vi "Measurement Logic.vi"() -> ()   [LabVIEW 2024, in "Frequency Response (Discrete Sweep).lvlib"]
uses:
  Frequency Response (Discrete Sweep).lvlib
  <vilib>/Plug-In SDKs/Measurements/Measure Call Context/Measure Call Context.lvclass
  Measurement Configuration.ctl
  Measurement Results.ctl
  <vilib>/gRPC/Generated APIs/ni/protobuf/types/RPC Messages/ni_protobuf_types_DoubleXYData.ctl
  C:/Program Files/NI/LVAddons/nisvt/1/examples/Sound and Vibration/Audio Measurements/subVIs/sv_AO Channel Configuration.ctl
  C:/Program Files/NI/LVAddons/nisvt/1/examples/Sound and Vibration/Audio Measurements/subVIs/sv_AI Channel Configuration.ctl
  <vilib>/addons/_NISVFA/_Shared subVIs/Controls/svc_Window.ctl
  <vilib>/addons/_NISVFA/_Generation/Signal Generation/SV Signal/SV Signal.lvclass/SV Signal.ctl
  <vilib>/addons/Sound and Vibration/svt_Level/SVL AC & DC Level (Time) (1 Ch).vi
  <vilib>/addons/_NISVFA/_Shared subVIs/Common/SV Append Data (1 Ch) (DBL).vi
  <vilib>/addons/_NISVFA/_Shared subVIs/Common/SV Append Data (N Ch) (DBL).vi
  <extravilib>/ChannelInstances/High Speed Stream-a[.](wfm(dbl))/_Read For Replicate.vi
  <vilib>/addons/_NISVFA/_Shared subVIs/Common/svc_Get SV Channel Info.vi
  <vilib>/Analysis/baseanly.llb/Mean.vi
  <vilib>/Analysis/baseanly.llb/Mean (DBL).vi
  <vilib>/addons/_NISVFA/_Shared subVIs/Windowing/svfa_Scaled Time Domain Window (Array).vi
  <extravilib>/ChannelInstances/Tag-bool/Write.vi
  <vilib>/DAQmx/read.llb/DAQmx Read.vi
  <vilib>/DAQmx/read.llb/DAQmx Read (Analog 1D Wfm NChan NSamp Duration).vi
  <extravilib>/ChannelInstances/High Speed Stream-a[.](wfm(dbl))/Write.vi
  <vilib>/DAQmx/write.llb/DAQmx Write.vi
  <vilib>/DAQmx/write.llb/DAQmx Write (Analog Wfm 1Chan NSamp).vi
  C:/Program Files/NI/LVAddons/nisvt/1/examples/Sound and Vibration/Audio Measurements/subVIs/sv_Synchronization Gatekeeper.vi
  <vilib>/Utility/error.llb/Clear Errors.vi
  C:/Program Files/NI/LVAddons/nisvt/1/examples/Sound and Vibration/Audio Measurements/subVIs/sv_Align and Parse for Stimulus Response.vi
  C:/Program Files/NI/LVAddons/nisvt/1/examples/Sound and Vibration/Audio Measurements/subVIs/sv_Synchronize Acquisition and Generation.vi
  C:/Program Files/NI/LVAddons/nisvt/1/examples/Sound and Vibration/Audio Measurements/subVIs/sv_Synchronize DSA AI and AO Tasks.vi
  <vilib>/addons/_NISVFA/_Shared subVIs/Common/svc_Unit Label to Engineering Units.vi
  <vilib>/addons/_NISVFA/_Shared subVIs/Common/svc_Engineering Units to Unit Label.vi
  <vilib>/addons/_NISVFA/_Spectrum Processing/subVIs/svfa_Spectrum Info Window to windowTd Type Def.vi
  <vilib>/Analysis/4window.llb/Force Window.vi
  <vilib>/Analysis/4window.llb/Force Window (DBL).vi
  <vilib>/Analysis/4window.llb/Exponential Window.vi
  <vilib>/Analysis/4window.llb/Exponential Window (DBL).vi
  <extravilib>/ChannelInstances/Tag-bool/Read With Abort.vi
  <extravilib>/ChannelInstances/Tag-bool/Write With Abort.vi
  C:/Program Files/NI/LVAddons/nisvt/1/examples/Sound and Vibration/Audio Measurements/subVIs/sv_Prepare Acquired Waveforms for Parsing.vi
  C:/Program Files/NI/LVAddons/nisvt/1/examples/Sound and Vibration/Audio Measurements/subVIs/sv_Timing for Stimulus Response Tasks.vi
  <vilib>/addons/_NISVFA/_Generation/Signal Generation/SV Signal/Read Total Samples.vi
  <vilib>/addons/_NISVFA/_Generation/Signal Generation/SV Signal/Write Leading Synchronization Pulse Enable.vi
  C:/Program Files/NI/LVAddons/nisvt/1/examples/Sound and Vibration/Audio Measurements/subVIs/sv_Synchronization Keymaster.vi
  C:/Program Files/NI/LVAddons/nisvt/1/examples/Sound and Vibration/Audio Measurements/subVIs/sv_Get Reference Clock.vi
  C:/Program Files/NI/LVAddons/nisvt/1/examples/Sound and Vibration/Audio Measurements/subVIs/sv_Synchronization Keymaster_GO.vi
  <extravilib>/ChannelInstances/Tag-c(ref(UserDefinedRefnumTag),t'Rendezvous RefNum')/Read With Abort.vi
  C:/Program Files/NI/LVAddons/nisvt/1/examples/Sound and Vibration/Audio Measurements/subVIs/sv_Align Waveforms by Leading Sync Pulse.vi
  <vilib>/addons/_NISVFA/_Generation/Signal Generation/SV Signal/Read Synchronization Pulse Waveform.vi
  <vilib>/addons/_NISVFA/_Shared subVIs/Common/svc_Check for Waveform Parameter Continuity (N Ch).vi
  C:/Program Files/NI/LVAddons/nisvt/1/examples/Sound and Vibration/Audio Measurements/subVIs/sv_Append Virtual Reference.vi
  <vilib>/addons/_NISVFA/_Generation/Signal Generation/SV Signal/Calculate Number of Remaining Samples.vi
  <extravilib>/ChannelInstances/Tag-c(ref(UserDefinedRefnumTag),t'Rendezvous RefNum')/Write.vi
  C:/Program Files/NI/LVAddons/nisvt/1/examples/Sound and Vibration/Audio Measurements/subVIs/sv_Measure Delay for Active and Idle Channels.vi
  <vilib>/addons/_NISVFA/_Generation/Signal Generation/SV Signal/Read Leading Synchronization Pulse Enable.vi
  <vilib>/addons/_NISVFA/_Generation/Signal Generation/SV Signal/Read Trailing Synchronization Pulse Enable.vi
  <vilib>/addons/_NISVFA/_Shared subVIs/Common/svc_Check for Waveform Parameter Continuity (no state).vi
  <vilib>/addons/_NISVFA/_Shared subVIs/Common/sv_Get NI Property Name String.vi
  <extravilib>/ChannelInstances/Tag-c(ref(UserDefinedRefnumTag),t'Rendezvous RefNum')/Write With Abort.vi
  <vilib>/addons/Sound and Vibration/svt_Calibration/SV Measure Delay and Polarity and Coherence (Nx1).vi
  C:/Program Files/NI/LVAddons/nisvt/1/examples/Sound and Vibration/Audio Measurements/subVIs/sv_Assign Delay to Idle Channels.vi
  <vilib>/addons/Sound and Vibration/svt_Calibration/SV Measure Delay and Polarity and Coherence.vi
  <vilib>/Analysis/_algsub.llb/Vector Norm.vi
  <vilib>/Analysis/_algsub.llb/Real Vector Norm.vi
  <vilib>/addons/_NISVFA/_Shared subVIs/Common/SV Get Data Subset.vi
  <vilib>/addons/_NISVFA/_Shared subVIs/Common/svc_Get Array Subset (Index).vi
  <vilib>/addons/_NISVFA/_Shared subVIs/Common/svc_Coerce Index and Length.vi
  <vilib>/addons/_NISVFA/_Shared subVIs/Common/svc_Conditional Merge Error.vi
  <vilib>/addons/_NISVFA/_Generation/Signal Generation/SV Discrete Sweep/SV Discrete Sweep.lvclass
  <extravilib>/ChannelInstances/Tag-bool/Instantiate.vi
  <extravilib>/ChannelInstances/High Speed Stream-a[.](wfm(dbl))/Instantiate.vi
  <vilib>/addons/_NISVFA/_Generation/Signal Generation/SV Discrete Sweep/Configure Frequency Sweep at Constant Amplitude.vi
  <vilib>/addons/_NISVFA/_Generation/Signal Generation/SV Signal/Write Ramp Parameters.vi
  <vilib>/addons/_NISVFA/_Generation/Signal Generation/SV Function/Write Pre-Measurement Settling Cycles.vi
  <vilib>/addons/_NISVFA/_Generation/Signal Generation/SV Function/Write Measurement Cycles.vi
  <vilib>/addons/_NISVFA/_Generation/Signal Generation/SV Signal/Write Measurement Duration.vi
  <extravilib>/ChannelInstances/High Speed Stream-a[.](wfm(dbl))/)Channel.vi
  <extravilib>/ChannelInstances/High Speed Stream-a[.](wfm(dbl))/Abort Signal/Init Signal.vi
  <vilib>/addons/_NISVFA/_Shared subVIs/Common/svc_Get Window Info.vi
  <vilib>/Analysis/0measdsp.llb/Scaled Time Domain Window.vi
  <vilib>/Analysis/0measdsp.llb/Scaled Time Domain Window (DBL).vi
  <vilib>/Utility/error.llb/Error Cluster From Error Code.vi
  <vilib>/Analysis/baseanly.llb/Std Deviation and Variance.vi
  <vilib>/addons/_NISVFA/_Shared subVIs/Common/svc_Caller VI Returned in Error Source.vi
  <vilib>/addons/Sound and Vibration/svt_Single Tone Measurements/SVT Gain and Phase (Time).vi
  <vilib>/addons/Sound and Vibration/svt_Distortion/SVT THD+N (Frequency) (1 Ch).vi
  <vilib>/addons/Sound and Vibration/svt_Distortion/SVT THD and Harmonic Components (Frequency) (1 Ch).vi
  <vilib>/addons/_NIFileIO/SV TDMS Write Waveform (N Ch).vi
  <extravilib>/ChannelInstances/Tag-bool/EndpointRead.vi
  <extravilib>/ChannelInstances/Tag-bool/Endpoint.vi
  <extravilib>/ChannelInstances/Tag-c(ref(UserDefinedRefnumTag),t'Rendezvous RefNum')/Instantiate.vi
  C:/Program Files/NI/LVAddons/nisvt/1/examples/Sound and Vibration/Audio Measurements/subVIs/sv_Configure AI Task.vi
  C:/Program Files/NI/LVAddons/nisvt/1/examples/Sound and Vibration/Audio Measurements/subVIs/sv_Configure AO Task.vi
  <vilib>/addons/_NISVFA/_Generation/Signal Generation/SV Signal/Read Sample Rate.vi
  <vilib>/addons/_NISVFA/_Generation/Signal Generation/SV Signal/Read Generation State.vi
  <vilib>/addons/_NISVFA/_Generation/Signal Generation/SV Signal/Read System Timing Model.vi
  <vilib>/DAQmx/configure/timing.llb/DAQmx Timing.vi
  <vilib>/DAQmx/configure/timing.llb/DAQmx Timing (Sample Clock).vi
  <vilib>/addons/_NISVFA/_Generation/Signal Generation/SV Signal/Write Sample Rate.vi
  <vilib>/DAQmx/configure/task.llb/DAQmx Stop Task.vi
  C:/Program Files/NI/LVAddons/nisvt/1/examples/Sound and Vibration/Audio Measurements/subVIs/sv_Get Bus Type and Product Type.vi
  <vilib>/DAQmx/configure/task.llb/DAQmx Control Task.vi
  <vilib>/Utility/rendezvs.llb/Create Rendezvous.vi
  <vilib>/Utility/rendezvs.llb/Wait at Rendezvous.vi
  <extravilib>/ChannelInstances/Tag-c(ref(UserDefinedRefnumTag),t'Rendezvous RefNum')/Endpoint.vi
  <vilib>/addons/Sound and Vibration/svt_DAQmx/subVIs/svl_Get Terminal Name with Device Prefix.vi
  <vilib>/DAQmx/configure/trigger.llb/DAQmx Trigger.vi
  <vilib>/DAQmx/configure/trigger.llb/DAQmx Start Trigger (Digital Edge).vi
  <vilib>/DAQmx/configure/task.llb/DAQmx Start Task.vi
  <extravilib>/ChannelInstances/Tag-c(ref(UserDefinedRefnumTag),t'Rendezvous RefNum')/EndpointRead.vi
  <vilib>/Utility/rendezvs.llb/Destroy Rendezvous.vi
  <vilib>/DAQmx/miscellaneous.llb/DAQmx Fill In Error Info.vi
  <vilib>/DAQmx/configure/task.llb/DAQmx Clear Task.vi
  <vilib>/Utility/LVClass/Get LV Class Name.vi
  <vilib>/addons/_NISVFA/_Generation/Signal Generation/SV Signal/Write System Timing Model.vi
  <vilib>/addons/_NISVFA/_Shared subVIs/Data Objects/Waveforms (DBL)/Write to Buffer.vi
  <vilib>/addons/_NISVFA/_Shared subVIs/Data Objects/Waveforms (DBL)/Read from Buffer.vi
  <vilib>/addons/_NISVFA/_Shared subVIs/Data Objects/Waveforms (DBL)/SV Read Newest Data.vi
  <vilib>/measure/maresamp.llb/Resample Waveforms (single shot).vi
  <vilib>/measure/maresamp.llb/Resample Waveform (single shot).vi
  <vilib>/addons/_NISVFA/_Shared subVIs/Common/svc_Check dt for Equal Sample Rates.vi
  <vilib>/Waveform/TSOps.llb/Timestamp Subtract.vi
  <vilib>/Analysis/2dsp.llb/CrossCorrelation.vi
  <vilib>/Analysis/2dsp.llb/1D Cross Correlation (DBL).vi
  <vilib>/addons/_NISVFA/_Shared subVIs/Common/svc_Fit Quadratic to Max Three Points in Array.vi
  <vilib>/addons/_NISVFA/_Shared subVIs/Common/SV Remove Delays (1,N) from Waveforms (N Ch) (DBL).vi
  <vilib>/addons/_NISVFA/_Shared subVIs/Common/SV Remove Delays from Waveforms.vi
  <vilib>/addons/_NISVFA/_Shared subVIs/Data Objects/Waveforms (DBL)/SV Read Next Measurement Data.vi
  <vilib>/DAQmx/configure/task.llb/DAQmx Wait Until Done.vi
  <extravilib>/ChannelInstances/Event Messenger-bool/Instantiate.vi
  <vilib>/addons/_NISVFA/_Generation/Signal Generation/SV Signal/SV Signal.lvclass
  <vilib>/gRPC/Generated APIs/ni/protobuf/types/ni.protobuf.types.lvlib
  <extravilib>/ChannelInstances/High Speed Stream-a[.](wfm(dbl)).lvlib
  C:/Program Files/NI/LVAddons/nisvt/1/examples/Sound and Vibration/SoundVib_Audio Examples.lvlib
  <vilib>/addons/Sound and Vibration/svt_Distortion/SoundVib_Distortion.lvlib
  <vilib>/addons/Sound and Vibration/svt_Single Tone Measurements/SoundVib_SingleTone.lvlib
panel:
  out "measurement results":T1={"current frequency"=0.0, "waveforms file path"="Empty", "reference RMS level"={"x_data"=[], "y_data"=[]}, "response RMS level"={"x_data"=[0.0], "y_data"=[0.0]}, "FRF magnitude"={"x_data"=[0.0], "y_data"=[0.0]}, "FRF phase"={"x_data"=[0.0], "y_data"=[]}, "THD"={"x_data"=[], "y_data"=[]}, "h2"={"x_data"=[], "y_data"=[]}, "h3"={"x_data"=[], "y_data"=[]}, "h4"={"x_data"=[], "y_data"=[]}, "h5"={"x_data"=[], "y_data"=[]}, "THDN"={"x_data"=[], "y_data"=[]}}
  in  "measurement configuration":T3={"sample rate"=51200.0, "ao stimulus channel"="Dev1/ao0", "ao range"=3.16, "ao terminal configuration"=-1, "ai reference channel"="Dev1/ai0", "ai ref range"=3.16, "ai reference terminal configuration"=-1, "ai response channel"="Dev1/ai1", "ai response range"=3.16, "ai response terminal configuration"=-1, "amplitude"=1.4142, "start frequency"=31.25, "stop frequency"=16000.0, "number of steps"=84, "profile"=enum."Logarithmic", "measurement time"=0.01, "measurement cycles"=10} {"measurement cycles" min=1; "measurement time" format="%#_4f s"; "stop frequency" format="%.2f Hz"; "start frequency" format="%.2f Hz"; "amplitude" format="%#_6f V"; "ai response range" format="± %#_6f V"; "ao range" format="± %#_4f V"; "sample rate" format="%#.2p Hz"}
  out "measure call context out":refnum<class "Measure Call Context.lvclass">
  in  "measure call context in":refnum<class "Measure Call Context.lvclass">
  out "error out":errorcluster
  in  "error in":errorcluster
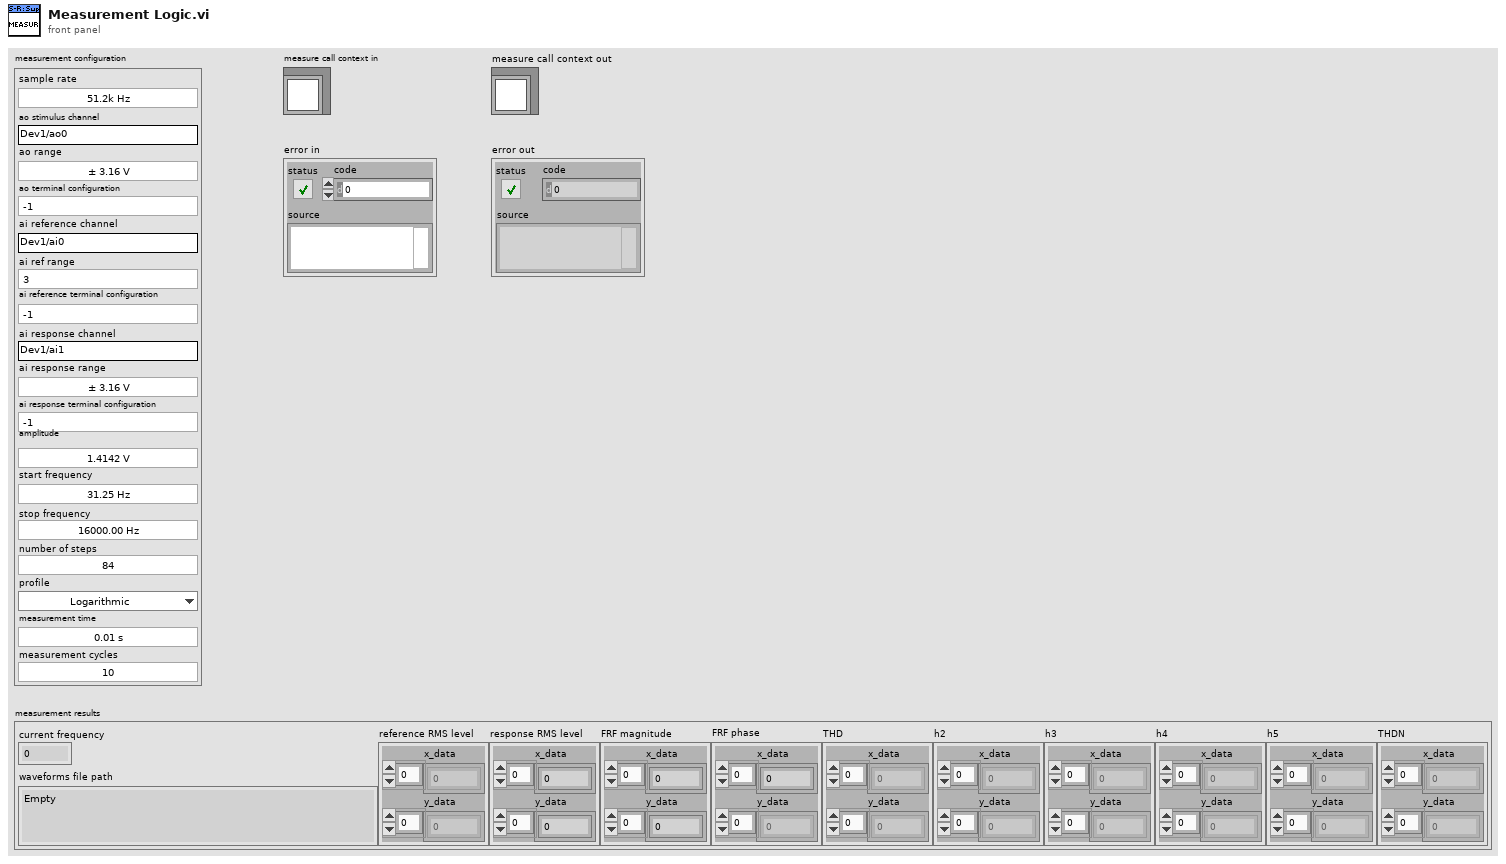
[diagram p1: front panel]
types:
  T1 = typedef "Frequency Response (Discrete Sweep).lvlib/Measurement Results.ctl" = cluster{"current frequency":dbl, "waveforms file path":string, "reference RMS level":T2, "response RMS level":T2, "FRF magnitude":T2, "FRF phase":T2, "THD":T2, "h2":T2, "h3":T2, "h4":T2, "h5":T2, "THDN":T2}
  T2 = typedef "ni.protobuf.types.lvlib/ni_protobuf_types_DoubleXYData.ctl" = cluster{"x_data":dbl[], "y_data":dbl[]}
  T3 = typedef "Frequency Response (Discrete Sweep).lvlib/Measurement Configuration.ctl" = cluster{"sample rate":dbl, "ao stimulus channel":string, "ao range":dbl, "ao terminal configuration":i32, "ai reference channel":string, "ai ref range":dbl, "ai reference terminal configuration":i32, "ai response channel":string, "ai response range":dbl, "ai response terminal configuration":i32, "amplitude":dbl, "start frequency":dbl, "stop frequency":dbl, "number of steps":i32, "profile":enum32{"Linear", "Logarithmic"}, "measurement time":dbl, "measurement cycles":i32}
  T4 = enum16{"open", "open or create", "create or replace", "create", "open (read-only)"}
  T5 = typedef "SoundVib_Audio Examples.lvlib/sv_AO Channel Configuration.ctl" = cluster{"DAQmx Channel":tag, "Max":dbl, "output terminal configuration":i32}
  T6 = cluster{"profile":enum16{"Linear", "Half cosine"}, "durations [s]":cluster{"ramp-up":dbl, "transition":dbl, "ramp-down":dbl}}
  T7 = typedef "SoundVib_Audio Examples.lvlib/sv_AI Channel Configuration.ctl" = cluster{"DAQmx Channel":tag, "Channel Type":u16, "Max":dbl, "Sensitivity":dbl, "Coupling":enum16{"AC", "DC"}, "excitation":enum16{"Off", "Min", "Max"}, "input terminal configuration":i32}
  T8 = typedef "High Speed Stream-a[.](wfm(dbl)).lvlib/)Channel.ctl" = refnum<queue>
  T9 = cluster{"start frequency":dbl, "stop frequency":dbl}
  T10 = cluster{"THD+N units":enum16{"dB", "linear ratio", "%"}, "detected fundamental amplitude units":enum16{"EU rms", "EU peak", "EU peak-peak"}}
  T11 = typedef "svc_Window.ctl" = u32
  T12 = cluster{"gain units":enum16{"dB", "linear ratio"}, "phase units":enum16{"deg", "rad"}, "detected tone stimulus amplitude units":enum16{"EU rms", "EU peak", "EU peak-peak"}, "detected tone response amplitude units":enum16{"EU rms", "EU peak", "EU peak-peak"}}
  T13 = cluster{"THD units":enum16{"dB", "linear ratio", "%"}, "harmonic component amplitude units":enum16{"EU rms", "EU peak", "EU peak-peak", "dB ref fund"}, "detected fundamental amplitude units":enum16{"EU rms", "EU peak", "EU peak-peak"}}
  T14 = typedef "svc_Spectrum Info.ctl" = cluster{"channel name":string, "description":string, "x-axis units":T15, "spectral info":cluster{"spectrum type":T16, "linear/dB":enum16{"linear", "dB"}, "window":u16, "window size":i32, "FFT size":i32}, "engineering units":T17, "custom label":string, "dB reference [EU]":dbl, "peak units":enum16{"rms", "peak", "peak-peak"}, "weighting filter":T18, "spectral density?":bool, "unit label":string, "spectrum skewed?":bool, "complimentary spectrum units":T19}
  T15 = typedef "svc_X-Axis Units.ctl" = u16
  T16 = typedef "svc_Spectrum Type.ctl" = enum16{"FFT Spectrum [complex]", "Amplitude [Magnitude]", "Power [Magnitude^2]", "Cross Spectrum [complex]", "Frequency Response [Complex]"}
  T17 = typedef "svc_Engineering Units Text Ring.ctl" = u16
  T18 = typedef "svc_Weighting Filter Text Ring.ctl" = u16
  T19 = typedef "svc_Complimentary Spectrum Units.ctl" = enum16{"none", "radians", "degrees", "cycles", "imaginary"}
  T20 = cluster{"complex spectrum response":cluster{"f0":dbl, "df":dbl, "complex spectrum":cdb[]}, "spectrum info":T14}
  T21 = typedef "Event Messenger-bool.lvlib/))Channel.ctl" = refnum<queue>
  T22 = typedef "Tag-bool.lvlib/))Channel.ctl" = refnum<queue>
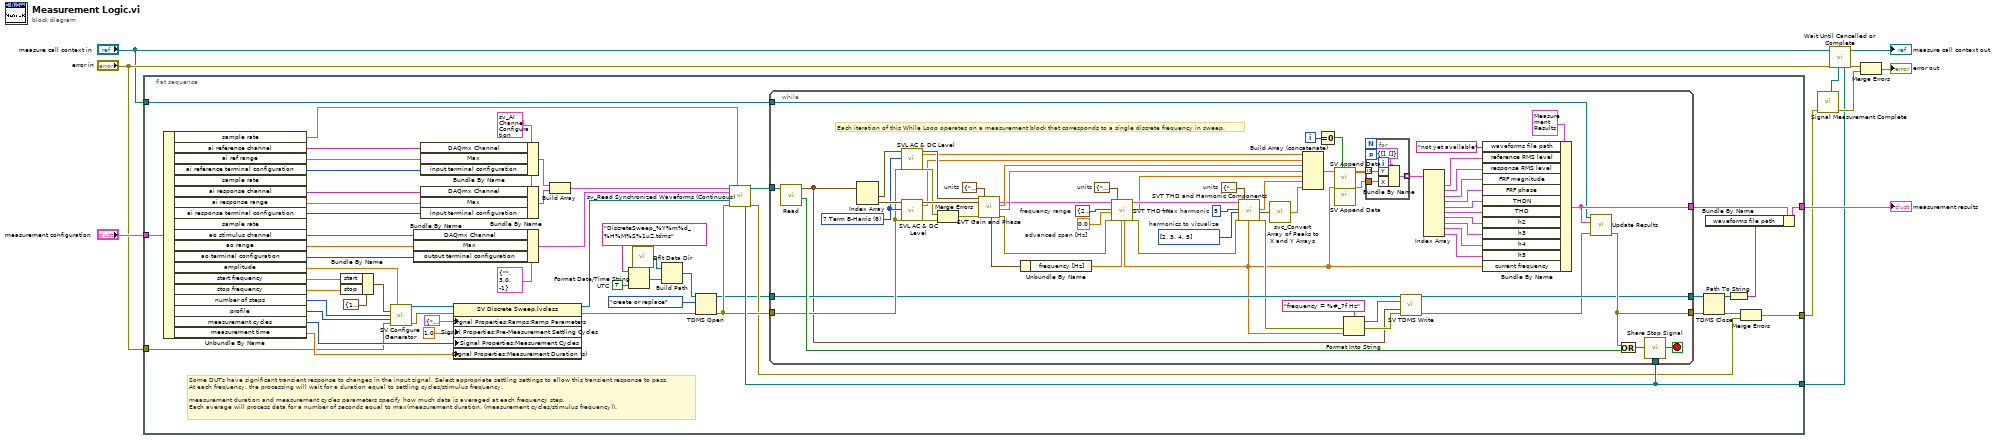
[diagram p0: block diagram]
diagram:
  n1 = flat-sequence {
    tunnel: "measurement configuration" -> [w64]
    tunnel: [w15] -> w10
    tunnel: "error in" -> [w31]
    tunnel: [w30] -> w7
    tunnel: w2 -> [w54]
    tunnel: "measure call context in" -> [w21]
    frame #0 {
      w12 = TRUE  # UTC
      w48 = T7 {"DAQmx Channel"="", "Channel Type"=0, "Max"=4.0, "Sensitivity"=1000.0, "Coupling"=enum."DC", "excitation"=enum."Off", "input terminal configuration"=-1} ("Channel Information")
      # "Some DUTs have significant transient response to changes in the input signal. Select appropriate settling settings to allow this transient response to pass.  \nAt each frequency, the processing will wait for a duration equal to settling cycles/stimulus frequency.\n\nmeasurement duration and measurement cycles parameters specify how much data is averaged at each frequency step.  \nEach average will process data for a number of seconds equal to max(measurement duration, (measurement cycles/stimulus frequency))."
      n2 = Unbundle By Name(w64) -> ("sample rate"=w53:dbl, "ai reference channel"=w52:string, "ai ref range"=w51:dbl, "ai reference terminal configuration"=w50:i32, "ai response channel"=w47:string, "ai response range"=w46:dbl, "ai response terminal configuration"=w45:i32, "ao stimulus channel"=w43:string, "ao range"=w42:dbl, "ao terminal configuration"=w41:i32, "amplitude"=w40:dbl, "start frequency"=w36:dbl, "stop frequency"=w35:dbl, "number of steps"=w38:i32, "profile"=w39:enum32{"Linear", "Logarithmic"}, "measurement cycles"=w33:i32, "measurement time"=w32:dbl)  [unwired: 2 out]
      n3 = Bundle By Name(cluster=cluster{"start":dbl, "stop":dbl} {"start"=100.0, "stop"=10000.0} ("frequency range [Hz]"), "start"=w36, "stop"=w35) -> (w34:cluster{"start":dbl, "stop":dbl})
      n4 = call-poly <vilib>:"SV Configure Generator.vi"("amplitude"=w40, "frequency range [Hz]"=w34, "number of steps"=w38, "profile"=w39, "error in (no error)"=w31) -> ("signal configuration"=w57:refnum<class "SV Discrete Sweep.lvclass">, "error out"=w56:errorcluster)  [unwired: 9 in]
      n5 = Bundle By Name(cluster=T5 {"DAQmx Channel"="", "Max"=3.0, "output terminal configuration"=-1} ("analog output channel"), "DAQmx Channel"=w43, "Max"=w42, "output terminal configuration"=w41) -> (w61:T5)
      n6 = Bundle By Name(cluster=w48, "DAQmx Channel"=w52, "Max"=w51, "input terminal configuration"=w50) -> (w49:T7)
      n7 = Bundle By Name(cluster=w48, "DAQmx Channel"=w47, "Max"=w46, "input terminal configuration"=w45) -> (w44:T7)
      n8 = property on="Property Node" class="SV Discrete Sweep.lvclass"(reference=w57, error in=w56, "Signal Properties:Ramps:Ramp Parameters"=T6 {"profile"=enum."Half cosine", "durations [s]"={"ramp-up"=0.05, "transition"=0.0, "ramp-down"=0.05}} ("Ramp Parameters"), "Signal Properties:Pre-Measurement Settling Cycles"=1.0 ("Pre-Measurement Settling Cycles"), "Signal Properties:Measurement Cycles"=w33, "Signal Properties:Measurement Duration (s)"=w32) -> (reference out=w58:refnum<class "SV Discrete Sweep.lvclass">, error out=w29:errorcluster)
      n9 = Build Array(w49, w44) -> (w62:T7[])
      n10 = Format Date/Time String(time format string (%c)="DiscreteSweep_%Y%m%d_%H%M%S%1uZ.tdms", UTC format=w12) -> (date/time string=w18:string)  [unwired: 1 in]
      n11 = call <vilib>:"Dflt Data Dir.vi"() -> ("App:Default Data Directory"=w19:path)
      n12 = Build Path(base path=w19, name or relative path=w18) -> (appended path=w17:path)
      n13 = TDMS Open(8:w29, 10:T4."create or replace" ("operation (0:open)"), 11:w17) -> (0:w28:errorcluster, 3:w24:refnum<k34>)  [unwired: 4 in]
      n14 = call "sv_Read Synchronized Waveforms (Continuous).vi"("ai channels"=w62, "sample rate (Hz)"=w53, "ao channel"=w61, "signal configuration"=w58, "error in"=w28, "stop channel"=w54) -> ("measurement channel"=w55:T8, "error out"=w27:errorcluster)  [unwired: 8 in]
      n15 = while {
        tunnel: [w125] -> w16
        tunnel: w55 -> [w128]
        tunnel: w54 -> [w127]
        tunnel: w28 -> [w76]
        tunnel: [w123] -> w26
        tunnel: w21 -> [w124]
        tunnel: w24 -> [w75]
        tunnel: [w74] -> w23
        i -> [w96]
        stop <- w126 stop-if-true
        w77 = 0.0  # advanced span [Hz]
        w91 = T9 {"start frequency"=20.0, "stop frequency"=20000.0}  # frequency range
        w92 = T10 {"THD+N units"=enum."dB", "detected fundamental amplitude units"=enum."EU rms"}  # units
        w101 = T11 8 items=["None"=0, "Hanning"=1, "Hamming"=2, "Blackman-Harris"=3, "Exact Blackman"=4, "Blackman"=5, "Flat Top"=6, "4 Term B-Harris "=7, "7 Term B-Harris"=8, "Low Sidelobe"=9, "Force"=64, "Exponential"=65, "Blackman Nuttall"=11, "Triangle"=30, "Bartlett-Hanning"=31, "Bohman"=32, "Parzen"=33, "Welch"=34, "Kaiser"=60, "Dolph-Chebyshev"=61, "Gaussian"=62] ("window")
        w118 = T12 {"gain units"=enum."dB", "phase units"=enum."deg", "detected tone stimulus amplitude units"=enum."EU rms", "detected tone response amplitude units"=enum."EU rms"}  # units
        w120 = T13 {"THD units"=enum."dB", "harmonic component amplitude units"=enum."dB ref fund", "detected fundamental amplitude units"=enum."EU peak"}  # units
        w119 = 5  # max harmonic
        w111 = i32[] [2, 3, 4, 5]  # harmonics to visualize
        # "This subVI created to clean up calling example diagram."
        # "Each iteration of this While Loop operates on a measurement block that corresponds to a single discrete frequency in sweep."
        n16 = call <extravilib>:"Read.vi"("channel"=w128) -> ("done?"=w122:bool, "element"=w68:waveform(dbl)[])  [unwired: 6 in, 3 out]
        n17 = Index Array(array=w68) -> (element #1=w103:waveform(dbl), element #2=w102:waveform(dbl))  [unwired: 2 in]
        n18 = call-poly <vilib>:"SVL AC & DC Level.vi"("scaled signal [EU]"=w103, "window"=w101, "error in (no error)"=w76) -> ("AC signal [EU]"=w117:waveform(dbl), "AC level [EU rms]"=w110:dbl, "error out"=w115:errorcluster)  [unwired: 11 in, 3 out]
        n19 = call-poly <vilib>:"SVL AC & DC Level.vi"("scaled signal [EU]"=w102, "window"=w101, "error in (no error)"=w76) -> ("AC signal [EU]"=w116:waveform(dbl), "AC level [EU rms]"=w109:dbl, "error out"=w114:errorcluster)  [unwired: 11 in, 3 out]
        n20 = Merge Errors(w115, w114) -> (w113:errorcluster)
        n21 = call-poly <vilib>:"SVT Gain and Phase.vi"("stimulus signal X [EUx]"=w117, "response signal Y [EUy]"=w116, "error in (no error)"=w113, "desired units"=w118) -> ("detected tone response"=w112:cluster{"frequency [Hz]":dbl, "amplitude":dbl}, "complex spectrum\nresponse Y"=w93:T20, "gain"=w108:dbl, "phase lag"=w107:dbl, "error out"=w66:errorcluster)  [unwired: 8 in, 3 out]
        n22 = Unbundle By Name(w112) -> ("frequency [Hz]"=w90:dbl)
        n23 = call-poly <vilib>:"SVT THD+N.vi"("complex spectrum"=w93, "frequency range"=w91, "advanced span [Hz]"=w77, "error in (no error)"=w66, "desired units"=w92, "expected fundamental frequency [Hz]"=w90) -> ("detected fundamental\nfrequency [Hz]"=w67:dbl, "dup complex spectrum"=w89:T20, "THD+N"=w88:dbl, "error out"=w65:errorcluster)  [unwired: 8 in, 2 out]
        n24 = call-poly <vilib>:"SVT THD and Harmonic Components.vi"("complex spectrum"=w89, "maximum harmonic"=w119, "harmonics to visualize"=w111, "error in (no error)"=w65, "desired units"=w120, "expected fundamental frequency [Hz]"=w67) -> ("THD"=w106:dbl, "harmonic components"=w105:cluster{"frequency [Hz]":dbl, "amplitude":dbl}[], "error out"=w70:errorcluster)  [unwired: 6 in, 5 out]
        n25 = call <vilib>:"svc_Convert Array of Peaks to X and Y Arrays.vi"("peaks"=w105) -> ("Y"=w94:dbl[])  [unwired: 3 in, 1 out]
        n26 = Build Array (concatenate)(w110, w109, w108, w107, w88, w106, w94) -> (w97:dbl[])
        n27 = Equal To 0?(x=w96) -> (x = 0?=w95:bool)
        n28 = call-poly <vilib>:"SV Append Data.vi"("reset (F)"=w95, "data in"=w97) -> ("appended data"=w98:dbl[][])  [unwired: 9 in]
        n29 = call-poly <vilib>:"SV Append Data.vi"("reset (F)"=w95, "data in"=w67) -> ("appended data"=w100:dbl[])  [unwired: 9 in]
        n30 = Format Into String(format string="frequency = %#_7f Hz", error in=w70, w67) -> (resulting string=w71:string, error out=w69:errorcluster)  [unwired: 1 in]
        n31 = for {
          tunnel: [w133] -> w99 mode=indexing
          tunnel: w98 -> [w132] mode=indexing
          workers-P: _ -> [_]
          tunnel: w100 -> [w130]
          n32 = Bundle By Name(cluster=cluster{"X":dbl[], "Y":dbl[]} {"X"=[], "Y"=[]} ("THD vs Amplitude"), "Y"=w132, "X"=w130) -> (w133:cluster{"X":dbl[], "Y":dbl[]})
        }
        n33 = call-poly <vilib>:"SV TDMS Write.vi"("tdms file"=w75, "group name in"=w71, "scaled signals"=w68, "error in"=w69) -> ("tdms file out"=w74:refnum<k34>, "error out"=w73:errorcluster)  [unwired: 8 in, 2 out]
        n34 = Index Array(array=w99) -> (element #1=w87:cluster{"X":dbl[], "Y":dbl[]}, element #2=w86:cluster{"X":dbl[], "Y":dbl[]}, element #3=w85:cluster{"X":dbl[], "Y":dbl[]}, element #4=w84:cluster{"X":dbl[], "Y":dbl[]}, element #5=w83:cluster{"X":dbl[], "Y":dbl[]}, element #6=w82:cluster{"X":dbl[], "Y":dbl[]}, element #7=w81:cluster{"X":dbl[], "Y":dbl[]}, element #8=w80:cluster{"X":dbl[], "Y":dbl[]}, element #9=w78:cluster{"X":dbl[], "Y":dbl[]}, element #10=w79:cluster{"X":dbl[], "Y":dbl[]})  [unwired: 10 in]
        n35 = Bundle By Name(cluster=T1 {"current frequency"=0.0, "waveforms file path"="Empty", "reference RMS level"={"x_data"=[], "y_data"=[]}, "response RMS level"={"x_data"=[], "y_data"=[0.0]}, "FRF magnitude"={"x_data"=[0.0], "y_data"=[0.0]}, "FRF phase"={"x_data"=[0.0], "y_data"=[]}, "THD"={"x_data"=[], "y_data"=[]}, "h2"={"x_data"=[], "y_data"=[]}, "h3"={"x_data"=[], "y_data"=[]}, "h4"={"x_data"=[], "y_data"=[]}, "h5"={"x_data"=[], "y_data"=[]}, "THDN"={"x_data"=[], "y_data"=[]}} ("Measurement Results"), "waveforms file path"="not yet available", "reference RMS level"=w87, "response RMS level"=w86, "FRF magnitude"=w85, "FRF phase"=w84, "THDN"=w83, "THD"=w82, "h2"=w81, "h3"=w80, "h4"=w78, "h5"=w79, "current frequency"=w67) -> (w125:T1)
        n36 = call <vilib>:"Update Results.vi"("error in"=w73, "measurement results"=w125, "measure call context in"=w124) -> ("error out"=w123:errorcluster)  [unwired: 7 in, 1 out]
        n37 = Or(x=w123, y=w122) -> (x .or. y?=w121:bool)
        n38 = call <vilib>:"Share Stop Signal.vi"("set stop (F)"=w121, "channel"=w127) -> ("stop"=w126:bool)
      }
      n39 = TDMS Close(8:w26, 11:w23) -> (0:w25:errorcluster, 3:w14:path)
      n40 = Path To String(path=w14) -> (string=w13:string)
      n41 = Bundle By Name(cluster=w16, "waveforms file path"=w13) -> (w15:T1)
      n42 = Merge Errors(w25, w27) -> (w30:errorcluster)
    }
  }
  n43 = call "Signal Measurement Complete.vi"("error in (no error)"=w7) -> ("error out"=w5:errorcluster, "done channel"=w6:T21)  [unwired: 9 in]
  n44 = call "Wait Until Cancelled or Complete.vi"("done channel"=w6, "error in (no error)"="error in", "measure call context in"="measure call context in") -> ("error out"=w4:errorcluster, "measure call context out"=→"measure call context out":refnum<class "Measure Call Context.lvclass">, "channel"=w2:T22)  [unwired: 6 in]
  n45 = Merge Errors(w4, w5) -> (→"error out":errorcluster)
  "measurement results" <- w10
